vi "GSI-HVSwitch2.ProcCases.vi"(0 "i ref in":refnum<vi>, 1 "selector":string, 2 "Data":T1, 3 "call cluster":T2={"Object"="", "Selector"="", "CallType"=enum."synchronous", "Async Object"="", "Async Selector"="", "Data Descriptor"="", "Data"=[], "Error #"=0, "Expire"=0}, 5 "error in (no error)":errorcluster) -> (14 "i ref out":refnum<vi>, 17 "answer cluster":T2={"Object"="", "Selector"="", "CallType"=enum."synchronous", "Async Object"="", "Async Selector"="", "Data Descriptor"="", "Data"=[], "Error #"=0, "Expire"=0}, 19 "error out":errorcluster)   [LabVIEW 2014, in "GSI-HVSwitch2.lvlib"]
doc: "This method is called by a process from within the default case in the event loop. The methods of a class that are linked to events will be called from THIS method. Add your code here."
uses:
  GSI-HVSwitch2.lvlib
  CS_Core/CSSystem/CoreDefs/CoreDefs.call_type.ctl
  CS_Core/BaseProcess/BaseProcess.descriptor string definition.ctl
  CS_Core/CSSystem/CoreDefs/CoreDefs.rawDataType.ctl
  CS_Core/CSSystem/CoreLib/CoreLib.string 2 byte array.vi
  CS_Core/CSSystem/CoreLib/CoreLib.byte array 2 double array.vi
  CS_Core/CSSystem/CoreLib/CoreLib.byte array 2 int.vi
  CS_Core/CSSystem/CoreLib/CoreLib.byte array 2 short.vi
  CS_Core/CSSystem/CoreLib/CoreLib.byte array 2 double.vi
  CS_Core/CSSystem/CoreLib/CoreLib.double 2 byte array.vi
  CS_Core/CSSystem/CoreLib/CoreLib.lvlib
  CS_Core/BaseProcess/BaseProcess.lvlib
  CS_Core/CSApplicationBaseClasses/PSChannelBase/PSChannelBase.lvlib
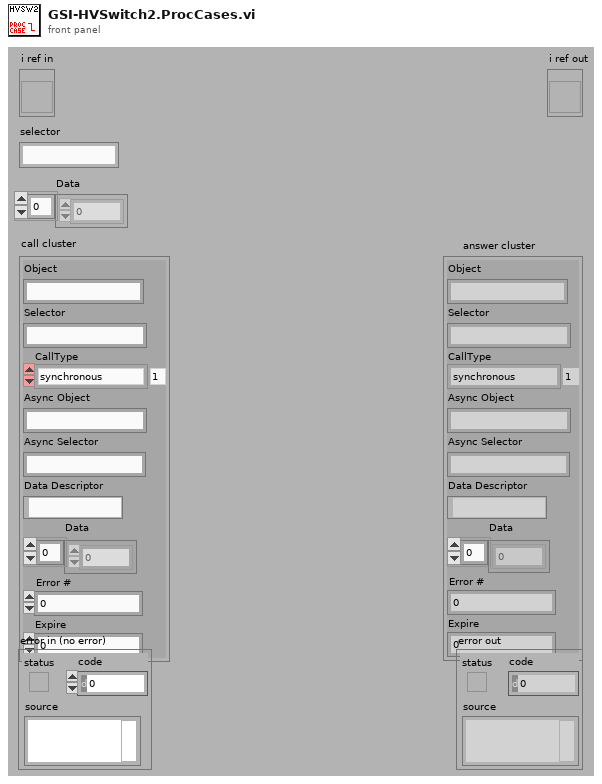
[diagram p1: front panel]
types:
  T1 = typedef "CoreDefs.rawDataType.ctl" = i8[]
  T2 = typedef "CoreDefs.call_type.ctl" = cluster{"Object":string, "Selector":string, "CallType":enum16{"simple", "synchronous", "asynchronous"}, "Async Object":string, "Async Selector":string, "Data Descriptor":T3, "Data":T1, "Error #":i32, "Expire":u32}
  T3 = typedef "BaseProcess.lvlib/BaseProcess.descriptor string definition.ctl" = string
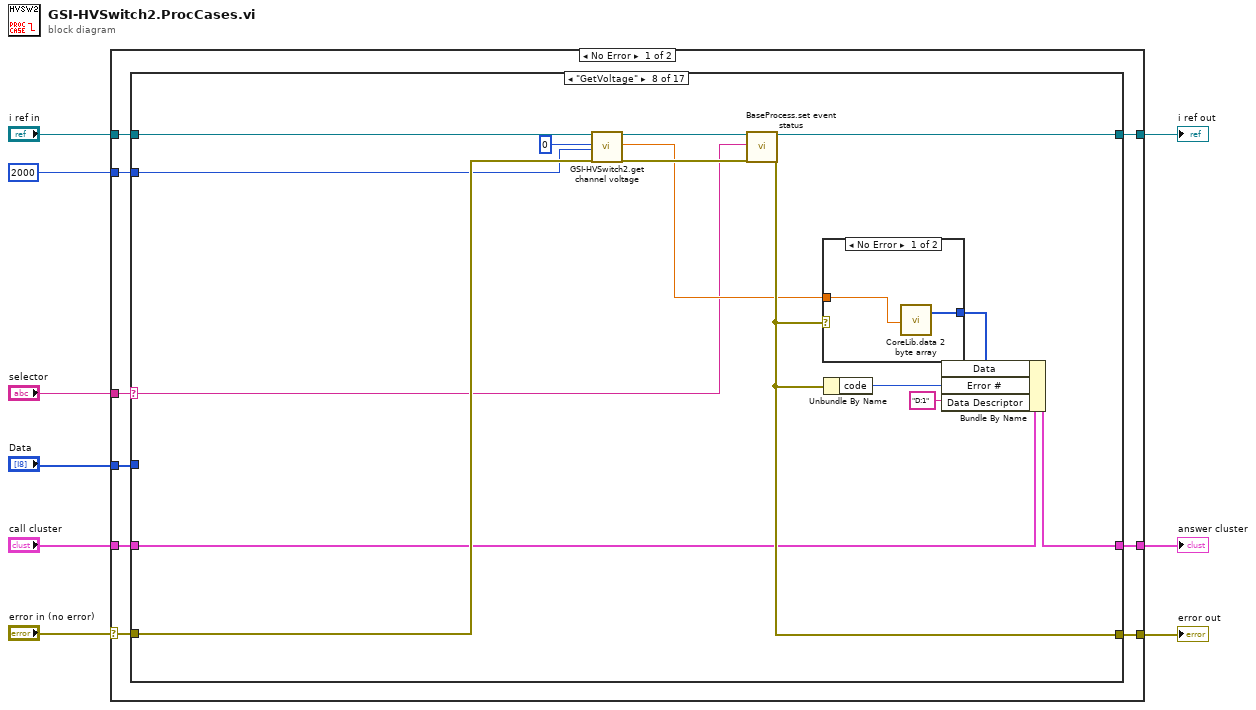
[diagram p0: block diagram]
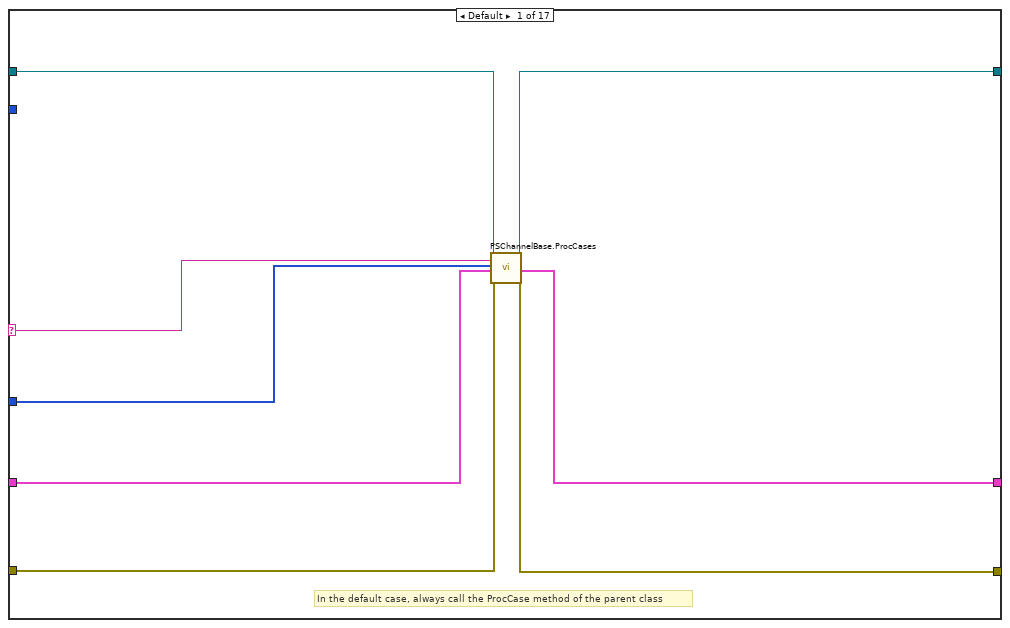
[diagram p2: hidden frame]
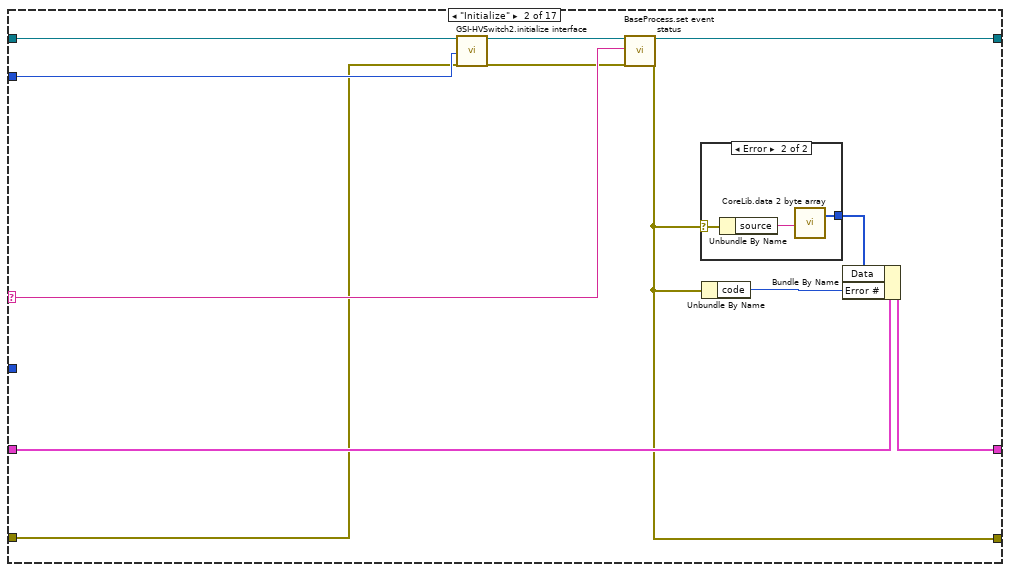
[diagram p3: hidden frame]
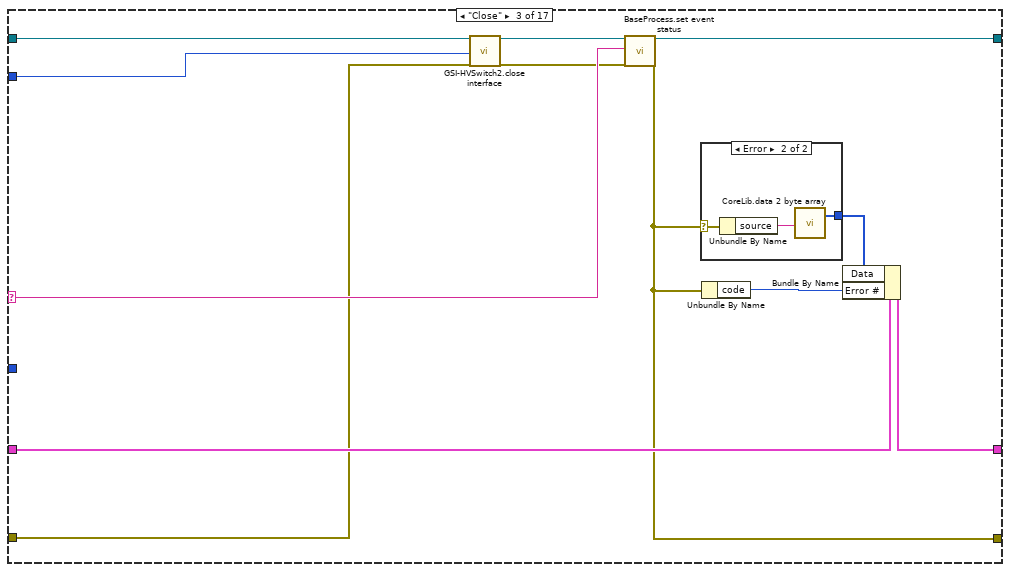
[diagram p5: hidden frame]
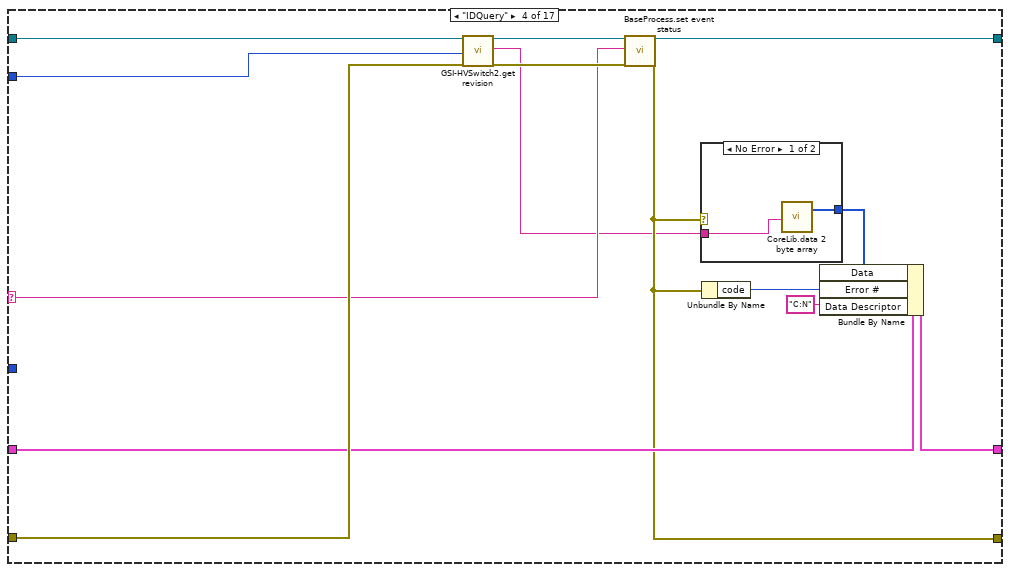
[diagram p7: hidden frame]
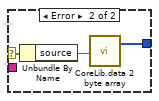
[diagram p8: hidden frame]
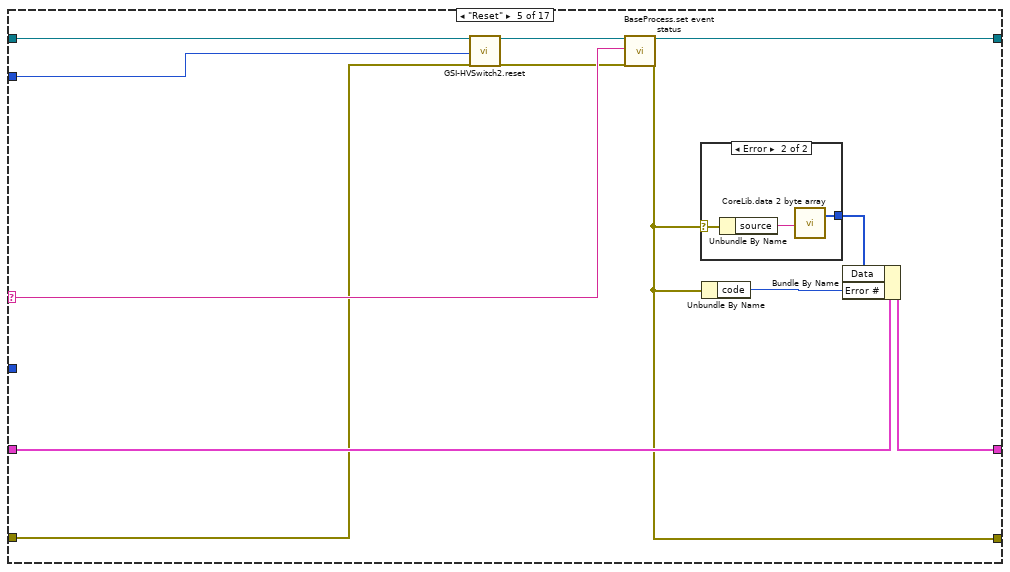
[diagram p9: hidden frame]
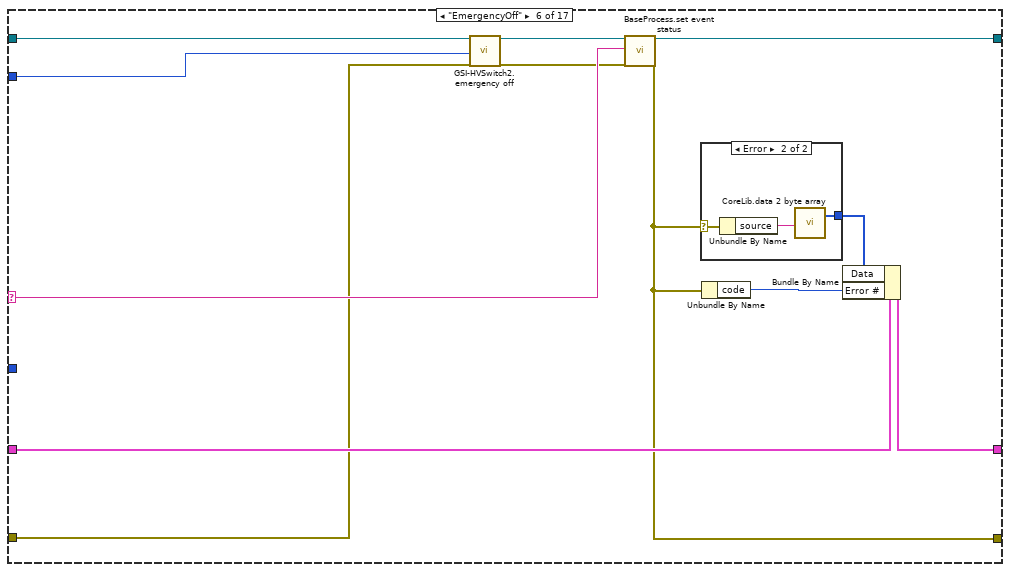
[diagram p11: hidden frame]
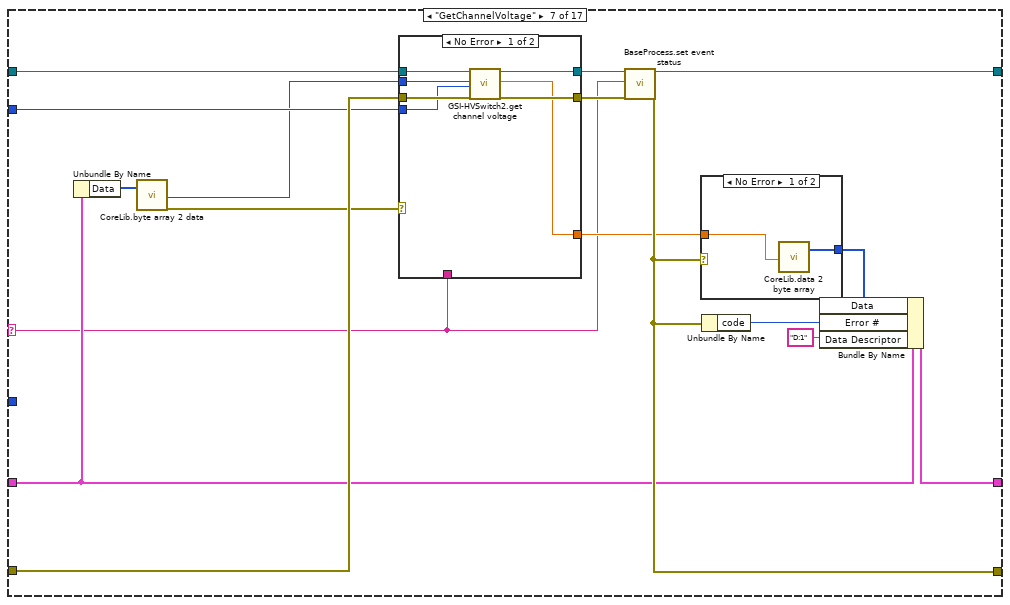
[diagram p13: hidden frame]
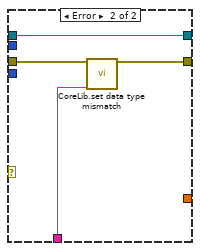
[diagram p14: hidden frame]
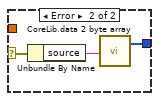
[diagram p15: hidden frame]
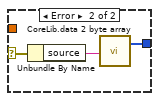
[diagram p16: hidden frame]
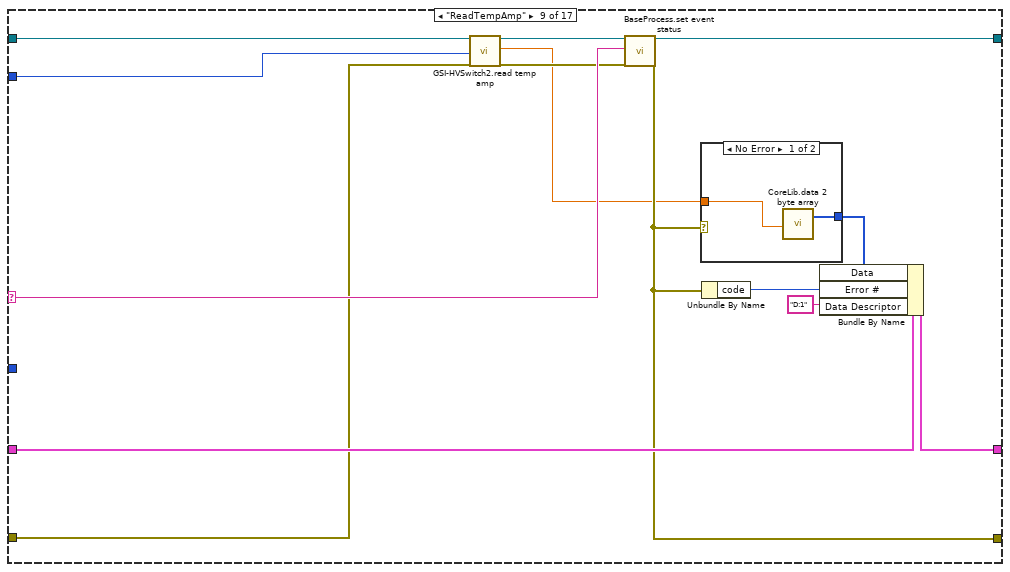
[diagram p17: hidden frame]
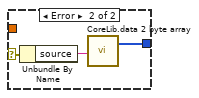
[diagram p18: hidden frame]
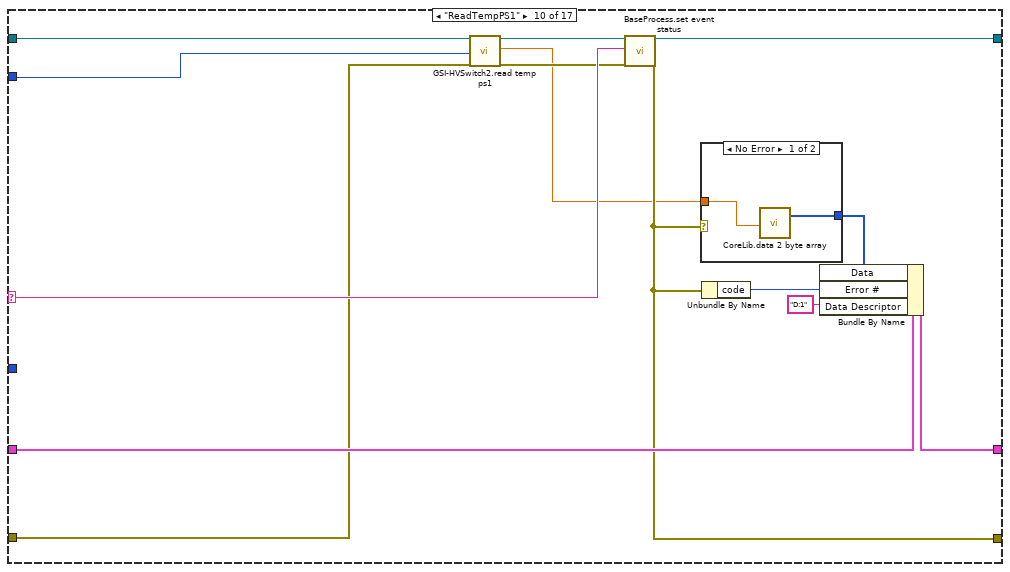
[diagram p19: hidden frame]
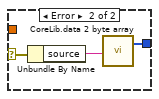
[diagram p20: hidden frame]
diagram:
  n1 = case shown="No Error" "error in (no error)" {
    selector: "error in (no error)" -> [w10 w397]
    tunnel: "selector" -> [w18 _]
    tunnel: [w17 w396] -> w8
    tunnel: "Data" -> [w16 _]
    tunnel: "call cluster" -> [w15 w396]
    tunnel: "i ref in" -> [w14 w395]
    tunnel: [w13 w395] -> w4
    tunnel: [w12 w397] -> w3
    tunnel: 2000 ("ms timeout (100)") -> [w11 _]
    frame No Error {
      n2 = case shown="\"GetVoltage\"" w18 {
        selector: w18 -> [w20 w33 w48 w61 w82 w97 w106 w140 w167 w186 w205 w221 w250 w282 w315 w344 w372]
        tunnel: w16 -> [w21 _ _ _ _ _ _ _ _ _ _ _ _ _ _ _ _]
        tunnel: w14 -> [w19 w28 w46 w70 w80 w95 w116 w147 w164 w183 w202 w230 w259 w291 w324 w353 w381]
        tunnel: [w26 w32 w47 w60 w81 w96 w118 w149 w166 w185 w204 w220 w249 w281 w314 w343 w371] -> w13
        tunnel: w15 -> [w22 w37 w52 w67 w86 w101 w110 w141 w171 w190 w209 w227 w256 w288 w321 w350 w378]
        tunnel: [w23 w36 w51 w66 w85 w100 w121 w152 w170 w189 w208 w226 w255 w287 w320 w349 w377] -> w17
        tunnel: w10 -> [w25 w27 w45 w69 w79 w94 w115 w146 w163 w182 w201 w229 w258 w290 w323 w352 w380]
        tunnel: [w24 w34 w49 w62 w83 w98 w119 w150 w168 w187 w206 w222 w251 w283 w316 w345 w373] -> w12
        tunnel: w11 -> [_ w29 w44 w59 w76 w91 w111 w142 w159 w178 w197 w219 w248 w280 w313 w342 w370]
        frame Default {
          # "In the default case, always call the ProcCase method of the parent class"
          n3 = call "PSChannelBase.ProcCases.vi"("i ref in"=w19, "selector"=w20, "Data"=w21, "call cluster"=w22, "error in (no error)"=w25) -> ("i ref out"=w26:refnum<vi>, "answer cluster"=w23:T2, "error out"=w24:errorcluster)  [unwired: 12 in]
        }
        frame "Initialize" {
          n4 = call "GSI-HVSwitch2.initialize interface.vi"("i ref in"=w28, "ms timeout (10000)"=w29, "error in (no error)"=w27) -> ("i ref out"=w30:refnum<vi>, "error out"=w31:errorcluster)  [unwired: 14 in, 1 out]
          n5 = call "BaseProcess.set event status.vi"("i ref in"=w30, "EventStatus"=w33, "error in (no error)"=w31) -> ("i ref out"=w32:refnum<vi>, "error out"=w34:errorcluster)  [unwired: 14 in, 1 out]
          n6 = case shown="Error" w34 {
            selector: w34 -> [_ w41]
            tunnel: [_ w39] -> w35
            frame No Error {
            }
            frame Error {
              n7 = Unbundle By Name(w41) -> ("source"=w40:string)
              n8 = call-poly "CoreLib.data 2 byte array.vi"("string"=w40) -> ("byteArray out"=w39:T1)  [unwired: 18 in]
            }
          }
          n9 = Unbundle By Name(w34) -> ("code"=w38:i32)
          n10 = Bundle By Name(cluster=w37, "Data"=w35, "Error #"=w38) -> (w36:T2)
        }
        frame "Close" {
          n11 = call "GSI-HVSwitch2.close interface.vi"("i ref in"=w46, "ms timeout (10000)"=w44, "error in (no error)"=w45) -> ("i ref out"=w42:refnum<vi>, "error out"=w43:errorcluster)  [unwired: 14 in, 1 out]
          n12 = call "BaseProcess.set event status.vi"("i ref in"=w42, "EventStatus"=w48, "error in (no error)"=w43) -> ("i ref out"=w47:refnum<vi>, "error out"=w49:errorcluster)  [unwired: 14 in, 1 out]
          n13 = case shown="Error" w49 {
            selector: w49 -> [_ w56]
            tunnel: [_ w54] -> w50
            frame No Error {
            }
            frame Error {
              n14 = Unbundle By Name(w56) -> ("source"=w55:string)
              n15 = call-poly "CoreLib.data 2 byte array.vi"("string"=w55) -> ("byteArray out"=w54:T1)  [unwired: 18 in]
            }
          }
          n16 = Unbundle By Name(w49) -> ("code"=w53:i32)
          n17 = Bundle By Name(cluster=w52, "Data"=w50, "Error #"=w53) -> (w51:T2)
        }
        frame "IDQuery" {
          n18 = call "GSI-HVSwitch2.get revision.vi"("i ref in"=w70, "ms timeout (10000)"=w59, "error in (no error)"=w69) -> ("i ref out"=w64:refnum<vi>, "revision"=w58:string, "error out"=w63:errorcluster)  [unwired: 12 in, 2 out]
          n19 = call "BaseProcess.set event status.vi"("i ref in"=w64, "EventStatus"=w61, "error in (no error)"=w63) -> ("i ref out"=w60:refnum<vi>, "error out"=w62:errorcluster)  [unwired: 14 in, 1 out]
          n20 = case shown="No Error" w62 {
            selector: w62 -> [_ w75]
            tunnel: [w72 w73] -> w65
            tunnel: w58 -> [w71 _]
            frame No Error {
              n21 = call-poly "CoreLib.data 2 byte array.vi"("string"=w71) -> ("byteArray out"=w72:T1)  [unwired: 18 in]
            }
            frame Error {
              n22 = Unbundle By Name(w75) -> ("source"=w74:string)
              n23 = call-poly "CoreLib.data 2 byte array.vi"("string"=w74) -> ("byteArray out"=w73:T1)  [unwired: 18 in]
            }
          }
          n24 = Unbundle By Name(w62) -> ("code"=w68:i32)
          n25 = Bundle By Name(cluster=w67, "Data"=w65, "Error #"=w68, "Data Descriptor"="C:N") -> (w66:T2)
        }
        frame "Reset" {
          n26 = call "GSI-HVSwitch2.reset.vi"("i ref in"=w80, "ms timeout (10000)"=w76, "error in (no error)"=w79) -> ("i ref out"=w78:refnum<vi>, "error out"=w77:errorcluster)  [unwired: 14 in, 1 out]
          n27 = call "BaseProcess.set event status.vi"("i ref in"=w78, "EventStatus"=w82, "error in (no error)"=w77) -> ("i ref out"=w81:refnum<vi>, "error out"=w83:errorcluster)  [unwired: 14 in, 1 out]
          n28 = case shown="Error" w83 {
            selector: w83 -> [_ w90]
            tunnel: [_ w88] -> w84
            frame No Error {
            }
            frame Error {
              n29 = Unbundle By Name(w90) -> ("source"=w89:string)
              n30 = call-poly "CoreLib.data 2 byte array.vi"("string"=w89) -> ("byteArray out"=w88:T1)  [unwired: 18 in]
            }
          }
          n31 = Unbundle By Name(w83) -> ("code"=w87:i32)
          n32 = Bundle By Name(cluster=w86, "Data"=w84, "Error #"=w87) -> (w85:T2)
        }
        frame "EmergencyOff" {
          n33 = call "GSI-HVSwitch2.emergency off.vi"("i ref in"=w95, "ms timeout (10000)"=w91, "error in (no error)"=w94) -> ("i ref out"=w93:refnum<vi>, "error out"=w92:errorcluster)  [unwired: 14 in, 1 out]
          n34 = call "BaseProcess.set event status.vi"("i ref in"=w93, "EventStatus"=w97, "error in (no error)"=w92) -> ("i ref out"=w96:refnum<vi>, "error out"=w98:errorcluster)  [unwired: 14 in, 1 out]
          n35 = case shown="Error" w98 {
            selector: w98 -> [_ w105]
            tunnel: [_ w103] -> w99
            frame No Error {
            }
            frame Error {
              n36 = Unbundle By Name(w105) -> ("source"=w104:string)
              n37 = call-poly "CoreLib.data 2 byte array.vi"("string"=w104) -> ("byteArray out"=w103:T1)  [unwired: 18 in]
            }
          }
          n38 = Unbundle By Name(w98) -> ("code"=w102:i32)
          n39 = Bundle By Name(cluster=w101, "Data"=w99, "Error #"=w102) -> (w100:T2)
        }
        frame "GetChannelVoltage" {
          n40 = Unbundle By Name(w110) -> ("Data"=w109:T1)
          n41 = call-poly "CoreLib.byte array 2 data.vi"("byteArray"=w109) -> ("i32"=w107:i32, "error out"=w108:errorcluster)  [unwired: 16 in, 1 out]
          n42 = case shown="No Error" w108 {
            tunnel: w116 -> [w129 w131]
            tunnel: w115 -> [w128 w133]
            tunnel: [w127 w131] -> w114
            tunnel: [w126 w132] -> w113
            tunnel: [w125 _] -> w112
            tunnel: w111 -> [w124 _]
            tunnel: w107 -> [w123 _]
            tunnel: w106 -> [_ w130]
            frame No Error {
              n43 = call "GSI-HVSwitch2.get channel voltage.vi"("i ref in"=w129, "channel"=w123, "ms timeout (10000)"=w124, "error in (no error)"=w128) -> ("i ref out"=w127:refnum<vi>, "ActVoltage"=w125:dbl, "error out"=w126:errorcluster)  [unwired: 12 in, 1 out]
            }
            frame Error {
              n44 = call "CoreLib.set data type mismatch.vi"("error in (no error)"=w133, "error source"=w130) -> ("error out"=w132:errorcluster)  [unwired: 17 in]
            }
          }
          n45 = call "BaseProcess.set event status.vi"("i ref in"=w114, "EventStatus"=w106, "error in (no error)"=w113) -> ("i ref out"=w118:refnum<vi>, "error out"=w119:errorcluster)  [unwired: 14 in, 1 out]
          n46 = case shown="No Error" w119 {
            selector: w119 -> [_ w138]
            tunnel: [w135 w136] -> w120
            tunnel: w112 -> [w134 _]
            frame No Error {
              n47 = call-poly "CoreLib.data 2 byte array.vi"("f64"=w134) -> ("byteArray out"=w135:T1)  [unwired: 18 in]
            }
            frame Error {
              n48 = Unbundle By Name(w138) -> ("source"=w137:string)
              n49 = call-poly "CoreLib.data 2 byte array.vi"("string"=w137) -> ("byteArray out"=w136:T1)  [unwired: 18 in]
            }
          }
          n50 = Unbundle By Name(w119) -> ("code"=w122:i32)
          n51 = Bundle By Name(cluster=w110, "Data"=w120, "Error #"=w122, "Data Descriptor"="D:1") -> (w121:T2)
        }
        frame "GetVoltage" {
          n52 = call "GSI-HVSwitch2.get channel voltage.vi"("i ref in"=w147, "channel"=0, "ms timeout (10000)"=w142, "error in (no error)"=w146) -> ("i ref out"=w145:refnum<vi>, "ActVoltage"=w143:dbl, "error out"=w144:errorcluster)  [unwired: 12 in, 1 out]
          n53 = call "BaseProcess.set event status.vi"("i ref in"=w145, "EventStatus"=w140, "error in (no error)"=w144) -> ("i ref out"=w149:refnum<vi>, "error out"=w150:errorcluster)  [unwired: 14 in, 1 out]
          n54 = case shown="No Error" w150 {
            selector: w150 -> [_ w158]
            tunnel: [w155 w156] -> w151
            tunnel: w143 -> [w154 _]
            frame No Error {
              n55 = call-poly "CoreLib.data 2 byte array.vi"("f64"=w154) -> ("byteArray out"=w155:T1)  [unwired: 18 in]
            }
            frame Error {
              n56 = Unbundle By Name(w158) -> ("source"=w157:string)
              n57 = call-poly "CoreLib.data 2 byte array.vi"("string"=w157) -> ("byteArray out"=w156:T1)  [unwired: 18 in]
            }
          }
          n58 = Unbundle By Name(w150) -> ("code"=w153:i32)
          n59 = Bundle By Name(cluster=w141, "Data"=w151, "Error #"=w153, "Data Descriptor"="D:1") -> (w152:T2)
        }
        frame "ReadTempAmp" {
          n60 = call "GSI-HVSwitch2.read temp amp.vi"("i ref in"=w164, "ms timeout (10000)"=w159, "error in (no error)"=w163) -> ("i ref out"=w162:refnum<vi>, "ActTempAmp"=w160:dbl, "error out"=w161:errorcluster)  [unwired: 13 in, 1 out]
          n61 = call "BaseProcess.set event status.vi"("i ref in"=w162, "EventStatus"=w167, "error in (no error)"=w161) -> ("i ref out"=w166:refnum<vi>, "error out"=w168:errorcluster)  [unwired: 14 in, 1 out]
          n62 = case shown="No Error" w168 {
            selector: w168 -> [_ w177]
            tunnel: [w174 w175] -> w169
            tunnel: w160 -> [w173 _]
            frame No Error {
              n63 = call-poly "CoreLib.data 2 byte array.vi"("f64"=w173) -> ("byteArray out"=w174:T1)  [unwired: 18 in]
            }
            frame Error {
              n64 = Unbundle By Name(w177) -> ("source"=w176:string)
              n65 = call-poly "CoreLib.data 2 byte array.vi"("string"=w176) -> ("byteArray out"=w175:T1)  [unwired: 18 in]
            }
          }
          n66 = Unbundle By Name(w168) -> ("code"=w172:i32)
          n67 = Bundle By Name(cluster=w171, "Data"=w169, "Error #"=w172, "Data Descriptor"="D:1") -> (w170:T2)
        }
        frame "ReadTempPS1" {
          n68 = call "GSI-HVSwitch2.read temp ps1.vi"("i ref in"=w183, "ms timeout (10000)"=w178, "error in (no error)"=w182) -> ("i ref out"=w181:refnum<vi>, "ActTempPS1"=w179:dbl, "error out"=w180:errorcluster)  [unwired: 13 in, 1 out]
          n69 = call "BaseProcess.set event status.vi"("i ref in"=w181, "EventStatus"=w186, "error in (no error)"=w180) -> ("i ref out"=w185:refnum<vi>, "error out"=w187:errorcluster)  [unwired: 14 in, 1 out]
          n70 = case shown="No Error" w187 {
            selector: w187 -> [_ w196]
            tunnel: [w193 w194] -> w188
            tunnel: w179 -> [w192 _]
            frame No Error {
              n71 = call-poly "CoreLib.data 2 byte array.vi"("f64"=w192) -> ("byteArray out"=w193:T1)  [unwired: 18 in]
            }
            frame Error {
              n72 = Unbundle By Name(w196) -> ("source"=w195:string)
              n73 = call-poly "CoreLib.data 2 byte array.vi"("string"=w195) -> ("byteArray out"=w194:T1)  [unwired: 18 in]
            }
          }
          n74 = Unbundle By Name(w187) -> ("code"=w191:i32)
          n75 = Bundle By Name(cluster=w190, "Data"=w188, "Error #"=w191, "Data Descriptor"="D:1") -> (w189:T2)
        }
        frame "ReadTempPS2" {
          n76 = call "GSI-HVSwitch2.read temp ps2.vi"("i ref in"=w202, "ms timeout (10000)"=w197, "error in (no error)"=w201) -> ("i ref out"=w200:refnum<vi>, "ActTempPS2"=w198:dbl, "error out"=w199:errorcluster)  [unwired: 13 in, 1 out]
          n77 = call "BaseProcess.set event status.vi"("i ref in"=w200, "EventStatus"=w205, "error in (no error)"=w199) -> ("i ref out"=w204:refnum<vi>, "error out"=w206:errorcluster)  [unwired: 14 in, 1 out]
          n78 = case shown="No Error" w206 {
            selector: w206 -> [_ w215]
            tunnel: [w212 w213] -> w207
            tunnel: w198 -> [w211 _]
            frame No Error {
              n79 = call-poly "CoreLib.data 2 byte array.vi"("f64"=w211) -> ("byteArray out"=w212:T1)  [unwired: 18 in]
            }
            frame Error {
              n80 = Unbundle By Name(w215) -> ("source"=w214:string)
              n81 = call-poly "CoreLib.data 2 byte array.vi"("string"=w214) -> ("byteArray out"=w213:T1)  [unwired: 18 in]
            }
          }
          n82 = Unbundle By Name(w206) -> ("code"=w210:i32)
          n83 = Bundle By Name(cluster=w209, "Data"=w207, "Error #"=w210, "Data Descriptor"="D:1") -> (w208:T2)
        }
        frame "SetHighVoltage" {
          n84 = Unbundle By Name(w227) -> ("Data"=w218:T1)
          n85 = call-poly "CoreLib.byte array 2 data.vi"("byteArray"=w218) -> ("d64"=w217:dbl, "error out"=w216:errorcluster)  [unwired: 16 in, 1 out]
          n86 = case shown="No Error" w216 {
            tunnel: [w238 w244] -> w224
            tunnel: w230 -> [w240 w244]
            tunnel: w229 -> [w239 w243]
            tunnel: [w237 w242] -> w223
            tunnel: w221 -> [_ w241]
            tunnel: w217 -> [w236 _]
            tunnel: w219 -> [w235 _]
            frame No Error {
              n87 = call "GSI-HVSwitch2.set channel voltage.vi"("i ref in"=w240, "nomVoltage"=w236, "channel"=0, "ms timeout (10000)"=w235, "error in (no error)"=w239) -> ("i ref out"=w238:refnum<vi>, "error out"=w237:errorcluster)  [unwired: 12 in, 1 out]
            }
            frame Error {
              n88 = call "CoreLib.set data type mismatch.vi"("error in (no error)"=w243, "error source"=w241) -> ("error out"=w242:errorcluster)  [unwired: 17 in]
            }
          }
          n89 = call "BaseProcess.set event status.vi"("i ref in"=w224, "EventStatus"=w221, "error in (no error)"=w223) -> ("i ref out"=w220:refnum<vi>, "error out"=w222:errorcluster)  [unwired: 14 in, 1 out]
          n90 = case shown="Error" w222 {
            selector: w222 -> [_ w233]
            tunnel: [_ w231] -> w225
            frame No Error {
            }
            frame Error {
              n91 = Unbundle By Name(w233) -> ("source"=w232:string)
              n92 = call-poly "CoreLib.data 2 byte array.vi"("string"=w232) -> ("byteArray out"=w231:T1)  [unwired: 18 in]
            }
          }
          n93 = Unbundle By Name(w222) -> ("code"=w228:i32)
          n94 = Bundle By Name(cluster=w227, "Data"=w225, "Error #"=w228) -> (w226:T2)
        }
        frame "SetLowVoltage" {
          n95 = Unbundle By Name(w256) -> ("Data"=w247:T1)
          n96 = call-poly "CoreLib.byte array 2 data.vi"("byteArray"=w247) -> ("d64"=w246:dbl, "error out"=w245:errorcluster)  [unwired: 16 in, 1 out]
          n97 = case shown="No Error" w245 {
            tunnel: [w267 w273] -> w253
            tunnel: w259 -> [w269 w273]
            tunnel: w258 -> [w268 w272]
            tunnel: [w266 w271] -> w252
            tunnel: w250 -> [_ w270]
            tunnel: w246 -> [w265 _]
            tunnel: w248 -> [w264 _]
            frame No Error {
              n98 = call "GSI-HVSwitch2.set channel voltage.vi"("i ref in"=w269, "nomVoltage"=w265, "channel"=1, "ms timeout (10000)"=w264, "error in (no error)"=w268) -> ("i ref out"=w267:refnum<vi>, "error out"=w266:errorcluster)  [unwired: 12 in, 1 out]
            }
            frame Error {
              n99 = call "CoreLib.set data type mismatch.vi"("error in (no error)"=w272, "error source"=w270) -> ("error out"=w271:errorcluster)  [unwired: 17 in]
            }
          }
          n100 = call "BaseProcess.set event status.vi"("i ref in"=w253, "EventStatus"=w250, "error in (no error)"=w252) -> ("i ref out"=w249:refnum<vi>, "error out"=w251:errorcluster)  [unwired: 14 in, 1 out]
          n101 = case shown="Error" w251 {
            selector: w251 -> [_ w262]
            tunnel: [_ w260] -> w254
            frame No Error {
            }
            frame Error {
              n102 = Unbundle By Name(w262) -> ("source"=w261:string)
              n103 = call-poly "CoreLib.data 2 byte array.vi"("string"=w261) -> ("byteArray out"=w260:T1)  [unwired: 18 in]
            }
          }
          n104 = Unbundle By Name(w251) -> ("code"=w257:i32)
          n105 = Bundle By Name(cluster=w256, "Data"=w254, "Error #"=w257) -> (w255:T2)
        }
        frame "SetChannelVoltage" {
          n106 = Unbundle By Name(w288) -> ("Data"=w275:T1)
          n107 = call-poly "CoreLib.byte array 2 data.vi"("byteArray"=w275) -> ("byteArray out"=w277:T1, "i32"=w274:i32, "error out"=w276:errorcluster)  [unwired: 16 in]
          n108 = call-poly "CoreLib.byte array 2 data.vi"("byteArray"=w277, "error in (no error)"=w276) -> ("d64"=w279:dbl, "error out"=w278:errorcluster)  [unwired: 15 in, 1 out]
          n109 = case shown="No Error" w278 {
            tunnel: [w299 w305] -> w285
            tunnel: w291 -> [w301 w305]
            tunnel: w290 -> [w300 w304]
            tunnel: [w298 w303] -> w284
            tunnel: w282 -> [_ w302]
            tunnel: w279 -> [w297 _]
            tunnel: w280 -> [w296 _]
            tunnel: w274 -> [w295 _]
            frame No Error {
              n110 = call "GSI-HVSwitch2.set channel voltage.vi"("i ref in"=w301, "nomVoltage"=w297, "channel"=w295, "ms timeout (10000)"=w296, "error in (no error)"=w300) -> ("i ref out"=w299:refnum<vi>, "error out"=w298:errorcluster)  [unwired: 12 in, 1 out]
            }
            frame Error {
              n111 = call "CoreLib.set data type mismatch.vi"("error in (no error)"=w304, "error source"=w302) -> ("error out"=w303:errorcluster)  [unwired: 17 in]
            }
          }
          n112 = call "BaseProcess.set event status.vi"("i ref in"=w285, "EventStatus"=w282, "error in (no error)"=w284) -> ("i ref out"=w281:refnum<vi>, "error out"=w283:errorcluster)  [unwired: 14 in, 1 out]
          n113 = case shown="Error" w283 {
            selector: w283 -> [_ w294]
            tunnel: [_ w292] -> w286
            frame No Error {
            }
            frame Error {
              n114 = Unbundle By Name(w294) -> ("source"=w293:string)
              n115 = call-poly "CoreLib.data 2 byte array.vi"("string"=w293) -> ("byteArray out"=w292:T1)  [unwired: 18 in]
            }
          }
          n116 = Unbundle By Name(w283) -> ("code"=w289:i32)
          n117 = Bundle By Name(cluster=w288, "Data"=w286, "Error #"=w289) -> (w287:T2)
        }
        frame "SetChannelOnOff" {
          n118 = Unbundle By Name(w321) -> ("Data"=w308:T1)
          n119 = call-poly "CoreLib.byte array 2 data.vi"("byteArray"=w308) -> ("byteArray out"=w310:T1, "i32"=w307:i32, "error out"=w309:errorcluster)  [unwired: 16 in]
          n120 = call-poly "CoreLib.byte array 2 data.vi"("byteArray"=w310, "error in (no error)"=w309) -> ("i16"=w312:i16, "error out"=w311:errorcluster)  [unwired: 15 in, 1 out]
          n121 = Not Equal To 0?(x=w312) -> (x != 0?=w306:bool)
          n122 = case shown="No Error" w311 {
            tunnel: [w332 w338] -> w318
            tunnel: w324 -> [w334 w338]
            tunnel: w323 -> [w333 w337]
            tunnel: [w331 w336] -> w317
            tunnel: w315 -> [_ w335]
            tunnel: w306 -> [w330 _]
            tunnel: w313 -> [w329 _]
            tunnel: w307 -> [w328 _]
            frame No Error {
              n123 = call "GSI-HVSwitch2.set channel onOff.vi"("i ref in"=w334, "on (FALSE)"=w330, "channel"=w328, "ms timeout (10000)"=w329, "error in (no error)"=w333) -> ("i ref out"=w332:refnum<vi>, "error out"=w331:errorcluster)  [unwired: 12 in, 1 out]
            }
            frame Error {
              n124 = call "CoreLib.set data type mismatch.vi"("error in (no error)"=w337, "error source"=w335) -> ("error out"=w336:errorcluster)  [unwired: 17 in]
            }
          }
          n125 = call "BaseProcess.set event status.vi"("i ref in"=w318, "EventStatus"=w315, "error in (no error)"=w317) -> ("i ref out"=w314:refnum<vi>, "error out"=w316:errorcluster)  [unwired: 14 in, 1 out]
          n126 = case shown="Error" w316 {
            selector: w316 -> [_ w327]
            tunnel: [_ w325] -> w319
            frame No Error {
            }
            frame Error {
              n127 = Unbundle By Name(w327) -> ("source"=w326:string)
              n128 = call-poly "CoreLib.data 2 byte array.vi"("string"=w326) -> ("byteArray out"=w325:T1)  [unwired: 18 in]
            }
          }
          n129 = Unbundle By Name(w316) -> ("code"=w322:i32)
          n130 = Bundle By Name(cluster=w321, "Data"=w319, "Error #"=w322) -> (w320:T2)
        }
        frame "SetOperationalMode" {
          n131 = Unbundle By Name(w350) -> ("Data"=w341:T1)
          n132 = call-poly "CoreLib.byte array 2 data.vi"("byteArray"=w341) -> ("i32"=w340:i32, "error out"=w339:errorcluster)  [unwired: 16 in, 1 out]
          n133 = case shown="No Error" w339 {
            tunnel: [w360 w366] -> w347
            tunnel: w353 -> [w362 w366]
            tunnel: w352 -> [w361 w365]
            tunnel: [w359 w364] -> w346
            tunnel: w344 -> [_ w363]
            tunnel: w342 -> [w358 _]
            tunnel: w340 -> [w357 _]
            frame No Error {
              n134 = call "GSI-HVSwitch2.set operational mode.vi"("i ref in"=w362, "mode"=w357, "ms timeout (10000)"=w358, "error in (no error)"=w361) -> ("i ref out"=w360:refnum<vi>, "error out"=w359:errorcluster)  [unwired: 13 in, 1 out]
            }
            frame Error {
              n135 = call "CoreLib.set data type mismatch.vi"("error in (no error)"=w365, "error source"=w363) -> ("error out"=w364:errorcluster)  [unwired: 17 in]
            }
          }
          n136 = call "BaseProcess.set event status.vi"("i ref in"=w347, "EventStatus"=w344, "error in (no error)"=w346) -> ("i ref out"=w343:refnum<vi>, "error out"=w345:errorcluster)  [unwired: 14 in, 1 out]
          n137 = case shown="Error" w345 {
            selector: w345 -> [_ w356]
            tunnel: [_ w354] -> w348
            frame No Error {
            }
            frame Error {
              n138 = Unbundle By Name(w356) -> ("source"=w355:string)
              n139 = call-poly "CoreLib.data 2 byte array.vi"("string"=w355) -> ("byteArray out"=w354:T1)  [unwired: 18 in]
            }
          }
          n140 = Unbundle By Name(w345) -> ("code"=w351:i32)
          n141 = Bundle By Name(cluster=w350, "Data"=w348, "Error #"=w351) -> (w349:T2)
        }
        frame "SetVoltageSteps" {
          n142 = Unbundle By Name(w378) -> ("Data"=w369:T1)
          n143 = call-poly "CoreLib.byte array 2 data.vi"("byteArray"=w369) -> ("[d64]"=w368:dbl[], "error out"=w367:errorcluster)  [unwired: 16 in, 1 out]
          n144 = case shown="No Error" w367 {
            tunnel: [w388 w394] -> w375
            tunnel: w381 -> [w390 w394]
            tunnel: w380 -> [w389 w393]
            tunnel: [w387 w392] -> w374
            tunnel: w372 -> [_ w391]
            tunnel: w370 -> [w386 _]
            tunnel: w368 -> [w385 _]
            frame No Error {
              n145 = call "GSI-HVSwitch2.set voltage steps.vi"("i ref in"=w390, "voltageSteps [V]"=w385, "ms timeout (10000)"=w386, "error in (no error)"=w389) -> ("i ref out"=w388:refnum<vi>, "error out"=w387:errorcluster)  [unwired: 13 in, 1 out]
            }
            frame Error {
              n146 = call "CoreLib.set data type mismatch.vi"("error in (no error)"=w393, "error source"=w391) -> ("error out"=w392:errorcluster)  [unwired: 17 in]
            }
          }
          n147 = call "BaseProcess.set event status.vi"("i ref in"=w375, "EventStatus"=w372, "error in (no error)"=w374) -> ("i ref out"=w371:refnum<vi>, "error out"=w373:errorcluster)  [unwired: 14 in, 1 out]
          n148 = case shown="Error" w373 {
            selector: w373 -> [_ w384]
            tunnel: [_ w382] -> w376
            frame No Error {
            }
            frame Error {
              n149 = Unbundle By Name(w384) -> ("source"=w383:string)
              n150 = call-poly "CoreLib.data 2 byte array.vi"("string"=w383) -> ("byteArray out"=w382:T1)  [unwired: 18 in]
            }
          }
          n151 = Unbundle By Name(w373) -> ("code"=w379:i32)
          n152 = Bundle By Name(cluster=w378, "Data"=w376, "Error #"=w379) -> (w377:T2)
        }
      }
    }
    frame Error {
    }
  }
  "answer cluster" <- w8
  "i ref out" <- w4
  "error out" <- w3
